vi "Close.vi"(8 "error in (no error)":errorcluster, 11 "connection ID":refnum<k16>) -> (0 "error out":errorcluster)   [LabVIEW 2018, in "Simple UDP Message.lvlib"]
uses:
  Simple UDP Message.lvlib
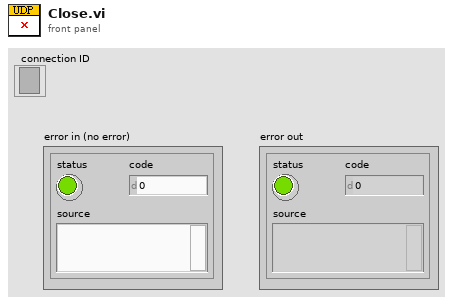
[diagram p1: front panel]
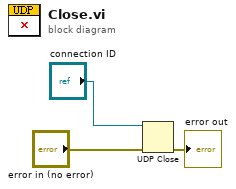
[diagram p0: block diagram]
diagram:
  n1 = UDP Close(connection ID="connection ID", 8:"error in (no error)") -> (error out=→"error out":errorcluster)  [unwired: 1 out]
